vi "EG_G5210 SetTrigMode.vi"(8 "error in (no error)":errorcluster, 10 "TrigMode":T1 items=["Reference", "External", "Asynchronous", "Ratio", "8F"], 11 "Ressource VISA":refnum<visa-resource-name>="GPIB0::8::INSTR") -> (0 "error out":errorcluster, 3 "Ressource VISA Out":refnum<visa-resource-name>="GPIB0::8::INSTR")   [LabVIEW 2010]
uses:
  <userlib>/EG_G 5210 LIA/TrigMode.ctl
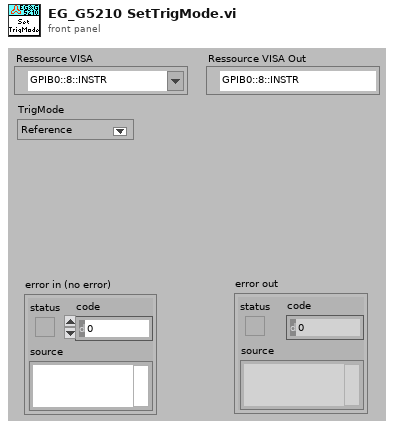
[diagram p1: front panel]
types:
  T1 = typedef "TrigMode.ctl" = u16
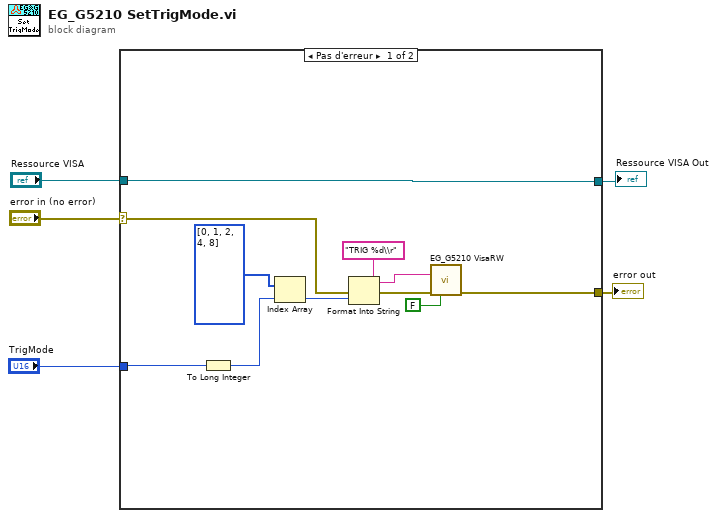
[diagram p0: block diagram]
diagram:
  n1 = case shown="Pas d'erreur" "error in (no error)" {
    selector: "error in (no error)" -> [w7 w18]
    tunnel: [w16 w18] -> w4
    tunnel: [w15 w17] -> w3
    tunnel: "Ressource VISA" -> [w15 w17]
    tunnel: "TrigMode" -> [w9 _]
    frame No Error {
      n2 = To Long Integer(number=w9) -> (32bit integer=w6:i32)
      n3 = Index Array(array=i32[] [0, 1, 2, 4, 8], index=w6) -> (element=w8:i32)
      n4 = Format Into String(format string="TRIG %d\\r" ("ChaineCom"), error in=w7, w8) -> (resulting string=w13:string, error out=w12:errorcluster)  [unwired: 1 in]
      n5 = call <userlib>:"EG_G5210 VisaRW.vi"("ChaineCom"=w13, "error in (no error)"=w12, "Lecture?(T)"=FALSE) -> ("error out"=w16:errorcluster)  [unwired: 9 in, 3 out]
    }
    frame Error {
    }
  }
  "error out" <- w4
  "Ressource VISA Out" <- w3
